vi "test_det.vi"() -> ()   [LabVIEW 2015]
uses:
  Classes/Detector/UV-VIS_AVANTES/def_parameters.ctl
  Classes/Detector/UV-VIS_AVANTES/UV-VIS_AVANTES.lvclass
panel:
  out "data":string
  out "unsigned byte array":u8[](array[numeric])
  out "parameters cluster":T1
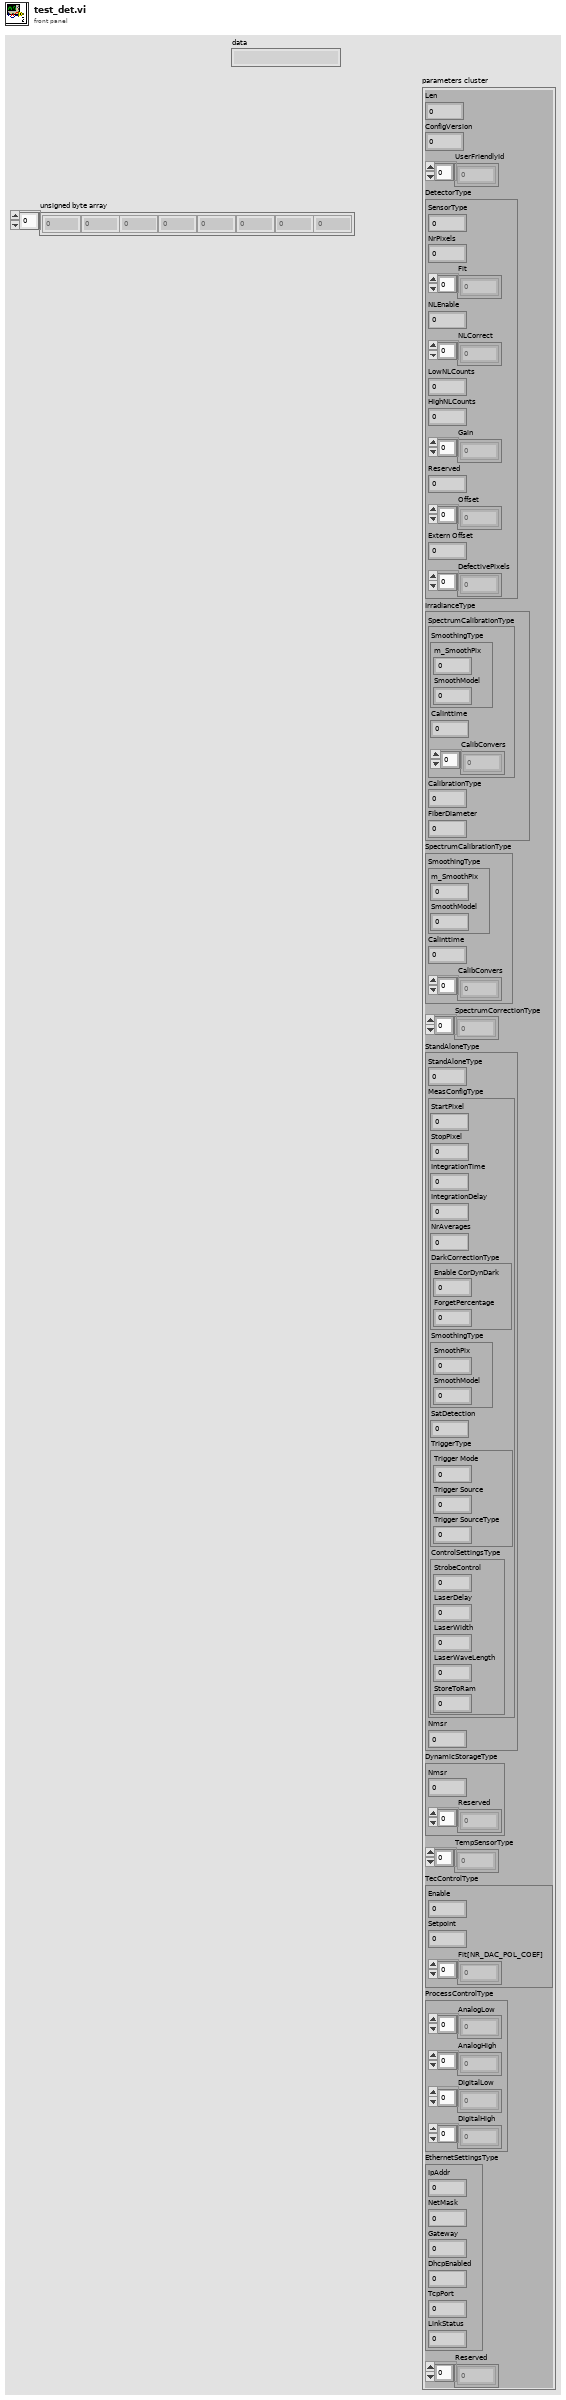
[diagram p1: front panel]
types:
  T1 = typedef "def_parameters.ctl" = cluster{"Len":u16, "ConfigVersion":u16, "UserFriendlyId":u8[], "DetectorType":cluster{"SensorType":u8, "NrPixels":u16, "Fit":sgl[], "NLEnable":u8, "NLCorrect":dbl[], "LowNLCounts":dbl, "HighNLCounts":dbl, "Gain":sgl[], "Reserved":sgl, "Offset":sgl[], "Extern Offset":sgl, "DefectivePixels":u16[]}, "IrradianceType":cluster{"SpectrumCalibrationType":cluster{"SmoothingType":cluster{"m_SmoothPix":u16, "SmoothModel":u8}, "CalInttime":sgl, "CalibConvers":sgl[]}, "CalibrationType":u8, "FiberDiameter":i32}, "SpectrumCalibrationType":cluster{"SmoothingType":cluster{"m_SmoothPix":u16, "SmoothModel":u8}, "CalInttime":sgl, "CalibConvers":sgl[]}, "SpectrumCorrectionType":sgl[], "StandAloneType":cluster{"StandAloneType":u8, "MeasConfigType":cluster{"StartPixel":u16, "StopPixel":u16, "IntegrationTime":sgl, "IntegrationDelay":u32, "NrAverages":u32, "DarkCorrectionType":cluster{"Enable CorDynDark":u8, "ForgetPercentage":u8}, "SmoothingType":cluster{"SmoothPix":u16, "SmoothModel":u8}, "SatDetection":u8, "TriggerType":cluster{"Trigger Mode":u8, "Trigger Source":u8, "Trigger SourceType":u8}, "ControlSettingsType":cluster{"StrobeControl":u16, "LaserDelay":u32, "LaserWidth":u32, "LaserWaveLength":sgl, "StoreToRam":u16}}, "Nmsr":i16}, "DynamicStorageType":cluster{"Nmsr":i32, "Reserved":u8[]}, "TempSensorType":sgl[], "TecControlType":cluster{"Enable":u8, "Setpoint":sgl, "Fit[NR_DAC_POL_COEF]":sgl[]}, "ProcessControlType":cluster{"AnalogLow":sgl[], "AnalogHigh":sgl[], "DigitalLow":sgl[], "DigitalHigh":sgl[]}, "EthernetSettingsType":cluster{"IpAddr":u32, "NetMask":u32, "Gateway":u32, "DhcpEnabled":u8, "TcpPort":u16, "LinkStatus":u8}, "Reserved":u8[]}
  T2 = enum16{"big-endian, network order", "native, host order", "little-endian"}
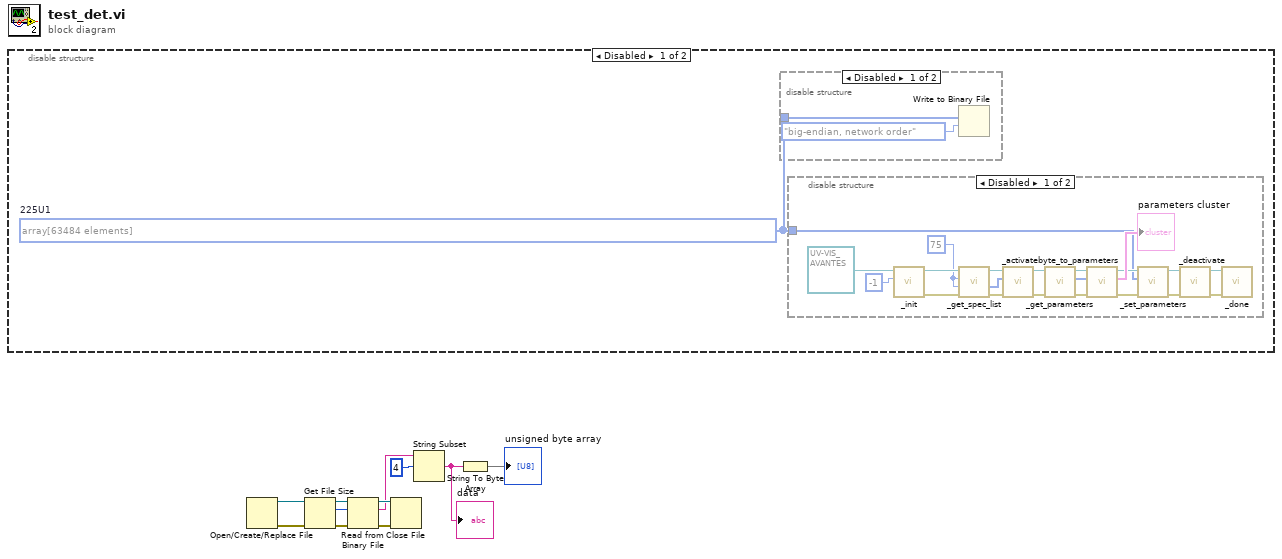
[diagram p0: block diagram]
diagram:
  n1 = disable-structure shown="Disabled" {
    frame Disabled {
      w12 = u8[] array[63484 elements]  # 225U1
      n2 = disable-structure shown="Disabled" {
        disable-tunnel: w12 -> [w14 _]
        frame Disabled {
          n3 = Write to Binary File(data=w14, 9:T2."big-endian, network order" ("byte order (0:big-endian, network order)")) -> ()  [unwired: 4 in, 3 out]
        }
        frame Enabled {
        }
      }
      n4 = disable-structure shown="Disabled" {
        disable-tunnel: w12 -> [w15 _]
        frame Disabled {
          w32 = 75 ("x")
          n5 = call "_init.vi"("a_Port"=i16 -1, "UV-VIS_AVANTES in"=refnum<class "UV-VIS_AVANTES.lvclass"> refnum ("UV-VIS_AVANTES.lvclass")) -> ("error out"=w29:errorcluster, "UV-VIS_AVANTES out"=w33:refnum<class "UV-VIS_AVANTES.lvclass">)  [unwired: 7 in, 1 out]
          n6 = call "_get_spec_list.vi"("error in (no error)"=w29, "RequiredSizeInput"=w32, "ListSizeInput"=w32, "UV-VIS_AVANTES in"=w33) -> ("error out"=w30:errorcluster, "List Output"=w31:u8[], "UV-VIS_AVANTES out"=w28:refnum<class "UV-VIS_AVANTES.lvclass">)  [unwired: 5 in]
          n7 = call "_activate.vi"("error in (no error)"=w30, "a_pDeviceId IN"=w31, "UV-VIS_AVANTES in"=w28) -> ("error out"=w26:errorcluster, "UV-VIS_AVANTES out"=w27:refnum<class "UV-VIS_AVANTES.lvclass">)  [unwired: 7 in]
          n8 = call "_get_parameters.vi"("error in (no error)"=w26, "UV-VIS_AVANTES in"=w27) -> ("error out"=w22:errorcluster, "DeviceParam"=w25:u8[], "UV-VIS_AVANTES out"=w24:refnum<class "UV-VIS_AVANTES.lvclass">)  [unwired: 7 in]
          n9 = call "byte_to_parameters.vi"("error in (no error)"=w22, "DeviceParam"=w25, "UV-VIS_AVANTES in"=w24) -> ("error out"=w17:errorcluster, "parameters cluster"=→"parameters cluster":T1, "UV-VIS_AVANTES out"=w19:refnum<class "UV-VIS_AVANTES.lvclass">)  [unwired: 6 in]
          n10 = call "_set_parameters.vi"("error in (no error)"=w17, "a_pDeviceParm"=w15, "UV-VIS_AVANTES in"=w19) -> ("error out"=w16:errorcluster, "UV-VIS_AVANTES out"=w18:refnum<class "UV-VIS_AVANTES.lvclass">)  [unwired: 6 in, 1 out]
          n11 = call "_deactivate.vi"("error in (no error)"=w16, "UV-VIS_AVANTES in"=w18) -> ("error out"=w21:errorcluster, "UV-VIS_AVANTES out"=w20:refnum<class "UV-VIS_AVANTES.lvclass">)  [unwired: 8 in]
          n12 = call "_done.vi"("error in (no error)"=w21, "UV-VIS_AVANTES in"=w20) -> ()  [unwired: 8 in, 2 out]
        }
        frame Enabled {
        }
      }
    }
    frame Enabled {
    }
  }
  n13 = Open/Create/Replace File() -> (refnum out=w2:refnum<file>, error out=w1:errorcluster)  [unwired: 6 in, 1 out]
  n14 = Get File Size(file=w2, error in=w1) -> (refnum out=w10:refnum<file>, size (in bytes)=w11:i64, 0:w9:errorcluster)
  n15 = Read from Binary File(8:w9, 10:w11, 11:w10) -> (0:w7:errorcluster, 2:w5:string, 3:w6:refnum<file>)  [unwired: 3 in, 1 out]
  n16 = Close File(refnum=w6, error in=w7) -> ()  [unwired: 2 out]
  n17 = String Subset(string=w5, offset (0)=4) -> (substring=w3:string)  [unwired: 1 in]
  "data" <- w3
  n18 = String To Byte Array(string=w3) -> (unsigned byte array=→"unsigned byte array":u8[])
